vi "Create.vi"(8 "error in (no error)":errorcluster) -> (0 "error out":errorcluster, 3 "Synchronous Request Callback Out":refnum<class "Synchronous Request Callback.lvclass">)   [LabVIEW 2020, in "Synchronous Request Callback.lvclass"]
uses:
  Synchronous Request Callback.lvclass
  Synchronous Request Callback.lvclass/Synchronous Request Callback.ctl
  Process/Protected/Messaging/Response Message Cluster.ctl
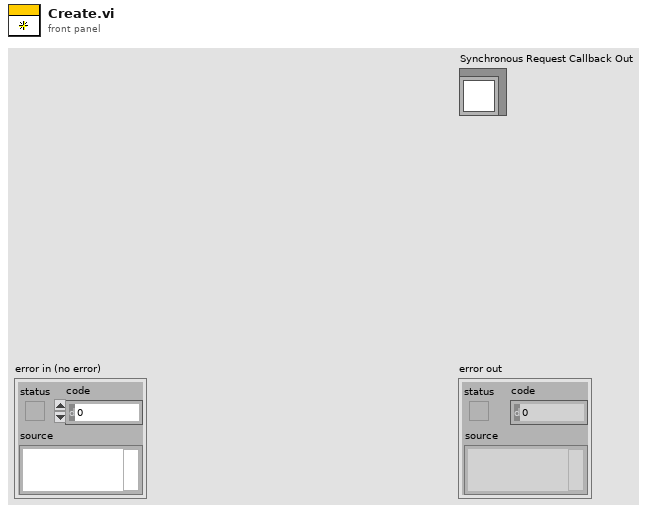
[diagram p1: front panel]
types:
  T1 = typedef "Synchronous Request Callback.lvclass/Response Message Cluster.ctl" = cluster{"Message":string, "Message Data":variant, "Error Out":errorcluster}
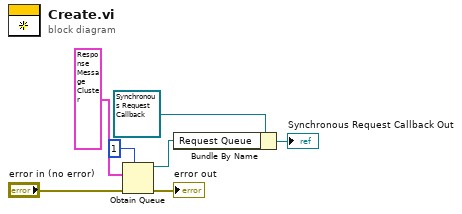
[diagram p0: block diagram]
diagram:
  n1 = Obtain Queue(max queue size (-1, unlimited)=1, element data type=T1 {"Message"="", "Message Data"=variant, "Error Out"={"status"=FALSE, "code"=0, "source"=""}} ("Message Cluster"), error in (no error)="error in (no error)") -> (queue out=w2:refnum<queue>, error out=→"error out":errorcluster)  [unwired: 2 in, 1 out]
  n2 = Bundle By Name(cluster=refnum<class "Synchronous Request Callback.lvclass"> refnum ("Synchronous Request Callback in"), "Request Queue"=w2) -> (→"Synchronous Request Callback Out":refnum<class "Synchronous Request Callback.lvclass">)
